vi "Pre Build.vi"(0 "Export In":refnum<class "Export.lvclass">) -> (4 "Export out":refnum<class "Export.lvclass">)   [LabVIEW 2017, in "CL_G3_VIComponentBuilder.lvlib" / "Export.lvclass"]
doc: "Executes any funtionality specified by the export before the export artifacts are created."
uses:
  Export.lvclass
  Export.lvclass/Export.ctl
  Accessors/Write Export Artifacts for SCC.vi
  Accessors/Write Export Operation Errors.vi
  Accessors/Read Export Build Specification.vi
  Accessors/Read Component Export Dir.vi
  Accessors/Read Export Operation Errors.vi
  CL_G3_VIComponentBuilder.lvlib
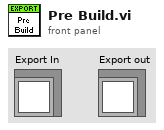
[diagram p1: front panel]
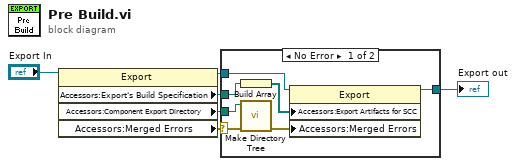
[diagram p0: block diagram]
diagram:
  n1 = property class="Export"(reference="Export In") -> (reference out=w4:refnum<class "Export.lvclass">, "Accessors:Export's Build Specification"=w2:path, "Accessors:Component Export Directory"=w1:path, "Accessors:Merged Errors"=w6:errorcluster)  [unwired: 1 in, 1 out]
  n2 = case shown="No Error" w6 {
    selector: w6 -> [w12 _]
    tunnel: w1 -> [w13 _]
    tunnel: w4 -> [w11 w14]
    tunnel: [w9 w14] -> w3
    tunnel: w2 -> [w8 _]
    frame No Error {
      n3 = Build Array(w8) -> (w7:path[])
      n4 = call "Make Directory Tree.vi"("error in (no error)"=w12, "Path"=w13) -> ("error out"=w10:errorcluster)  [unwired: 8 in, 1 out]
      n5 = property class="Export"(reference=w11, "Accessors:Export Artifacts for SCC"=w7, "Accessors:Merged Errors"=w10) -> (reference out=w9:refnum<class "Export.lvclass">)  [unwired: 1 in, 1 out]
    }
    frame Error {
    }
  }
  "Export out" <- w3
